vi "LC-MISDK_UserCalibration_TypeofCalib.vi"(0 "Cluster入力":refnum<vi>, 1 "Bool refnum 3":refnum<vi>, 2 "Clust refnum 4":refnum<vi>, 3 "Bool refnum 2":refnum<vi>, 4 "Clust refnum 5":refnum<vi>, 6 "Clust refnum 3":refnum<vi>, 7 "Clust refnum 6":refnum<vi>, 8 "Bool refnum 4":refnum<vi>, 9 "Clust refnum 7":refnum<vi>, 10 "Clust refnum入力":refnum<vi>, 11 "Clust refnum 8":refnum<vi>, 12 "Type of Calibration":enum32{"Single-Point", "RGB", "WRGB"}(ring), 13 "Bool refnum":refnum<vi>) -> ()   [LabVIEW 2015]
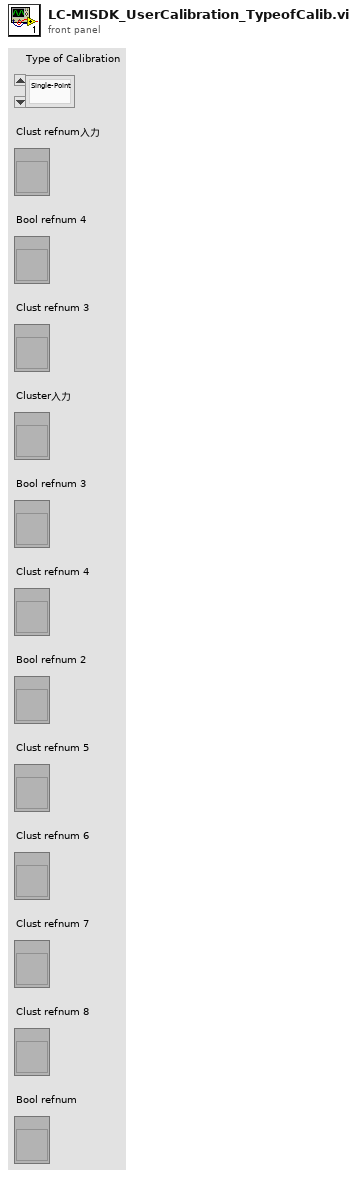
[diagram p1: front panel]
types:
  T1 = enum8{"Enabled", "Disabled", "Disabled and Grayed Out"}
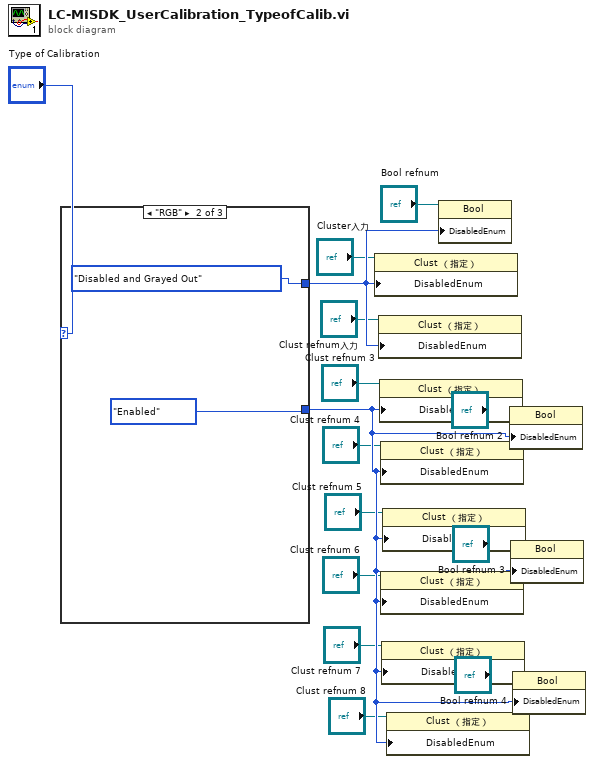
[diagram p0: block diagram]
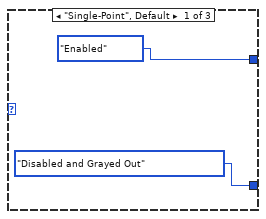
[diagram p2: hidden frame]
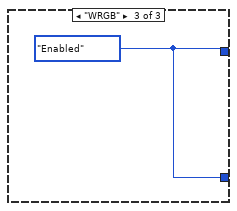
[diagram p3: hidden frame]
diagram:
  n1 = case shown="\"RGB\"" "Type of Calibration" {
    tunnel: [T1."Enabled" ("無効") T1."Disabled and Grayed Out" ("無効") w20] -> w14
    tunnel: [T1."Disabled and Grayed Out" ("無効") T1."Enabled" ("無効") w20] -> w15
    frame "Single-Point", Default {
    }
    frame "RGB" {
    }
    frame "WRGB" {
      w20 = T1."Enabled" ("無効")
    }
  }
  n2 = property on="プロパティノード" class="Clust （指定）"(reference="Cluster入力", "DisabledEnum"=w14) -> ()  [unwired: 1 in, 2 out]
  n3 = property on="プロパティノード" class="Clust （指定）"(reference="Clust refnum入力", "DisabledEnum"=w14) -> ()  [unwired: 1 in, 2 out]
  n4 = property on="プロパティノード" class="Clust （指定）"(reference="Clust refnum 3", "DisabledEnum"=w15) -> ()  [unwired: 1 in, 2 out]
  n5 = property on="プロパティノード" class="Clust （指定）"(reference="Clust refnum 4", "DisabledEnum"=w15) -> ()  [unwired: 1 in, 2 out]
  n6 = property on="プロパティノード" class="Clust （指定）"(reference="Clust refnum 6", "DisabledEnum"=w15) -> ()  [unwired: 1 in, 2 out]
  n7 = property on="プロパティノード" class="Clust （指定）"(reference="Clust refnum 7", "DisabledEnum"=w15) -> ()  [unwired: 1 in, 2 out]
  n8 = property on="プロパティノード" class="Clust （指定）"(reference="Clust refnum 5", "DisabledEnum"=w15) -> ()  [unwired: 1 in, 2 out]
  n9 = property on="プロパティノード" class="Clust （指定）"(reference="Clust refnum 8", "DisabledEnum"=w15) -> ()  [unwired: 1 in, 2 out]
  n10 = property on="プロパティノード" class="Bool"(reference="Bool refnum", "DisabledEnum"=w14) -> ()  [unwired: 1 in, 2 out]
  n11 = property on="プロパティノード" class="Bool"(reference="Bool refnum 2", "DisabledEnum"=w15) -> ()  [unwired: 1 in, 2 out]
  n12 = property on="プロパティノード" class="Bool"(reference="Bool refnum 3", "DisabledEnum"=w15) -> ()  [unwired: 1 in, 2 out]
  n13 = property on="プロパティノード" class="Bool"(reference="Bool refnum 4", "DisabledEnum"=w15) -> ()  [unwired: 1 in, 2 out]
